vi "Task 9 basic VI.vi"(0 "AE State":T2=enum."Open camera", 1 "error in (no error)":errorcluster) -> (2 "State done?":bool, 3 "Colour output boolean cluster":T1, 4 "error out":errorcluster)   [LabVIEW 2018]
uses:
  Task 9 Sates.ctl
  Modified webcam FGV/Webcam AE.ctl
  <vilib>/userdefined/High Color/IMAQdx.ctl
  I2C Master VI/Arduino_Interfacing.ctl
  I2C Master VI/I2C_MASTER_WRITE_NEW Type Def.ctl
  Elasped Timer/Elapsed timer control.ctl
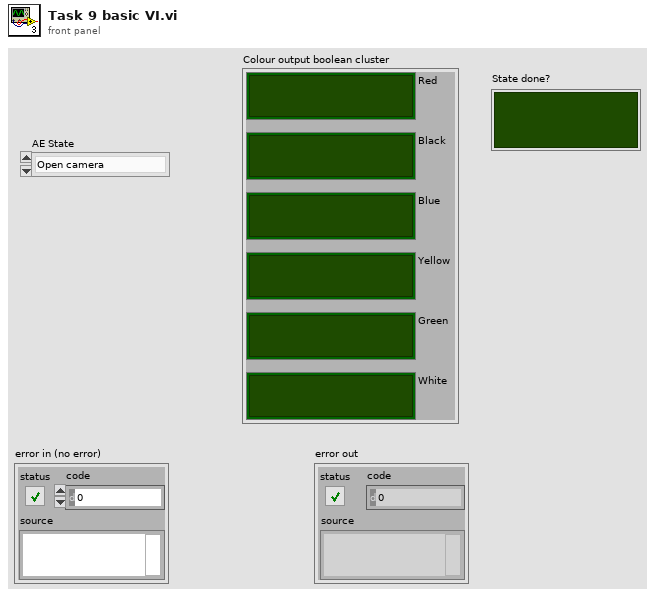
[diagram p1: front panel]
types:
  T1 = cluster{"Red":bool, "Black":bool, "Blue":bool, "Yellow":bool, "Green":bool, "White":bool}
  T2 = typedef "Task 9 Sates.ctl" = enum16{"Initialize", "Open camera", "Move Arm", "Set timer", "Capture images", "Close camera", "Process colour", "Dispose camera buffer"}
  T3 = typedef "Webcam AE.ctl" = enum16{"Initialize Camera", "Open Camera", "Continuous Acquisition", "Close Camera", "Retrieve Image", "Dispose Camera Image Buffer"}
  T4 = typedef "IMAQdx.ctl" = refnum<k21>
  T5 = typedef "I2C_MASTER_WRITE_NEW Type Def.ctl" = enum16{"Ultrasonic sensors", "Stepper origin", "zStepper 13.3k", "zStepper 13k", "zStepper 12k", "zStepper 11k", "zStepper 10k", "zStepper 9k", "zStepper 8k", "zStepper 7k", "zStepper 6k", "zStepper 5k", "zStepper 4k", "zStepper 3k", "zStepper 2k", "zStepper 1k", "zStepper 900", "zStepper 800", "zStepper 700", "zStepper 600", "zStepper 500", "zStepper 400", "zStepper 300", "zStepper 200", "zStepper 100", "zStepper 0", "yStepper control", "Open Claw", "Close Claw", "Soft Reset"}
  T6 = typedef "Arduino_Interfacing.ctl" = enum16{"Initialize", "Write to Arduino", "Read From Arduino"}
  T7 = typedef "Elapsed timer control.ctl" = enum16{"Start", "Pause", "Initialize"}
  T8 = cluster{"Arduino State":u8, "Rotary Switch":u8, "PING A":u8, "PING B":u8, "PING C":u8, "PING D":u8, "y Stepper Position":u8, "z Stepper Position":u8, "Data Out[8]":u8}
  T9 = typedef "IMAQ Image.ctl" = refnum<image>
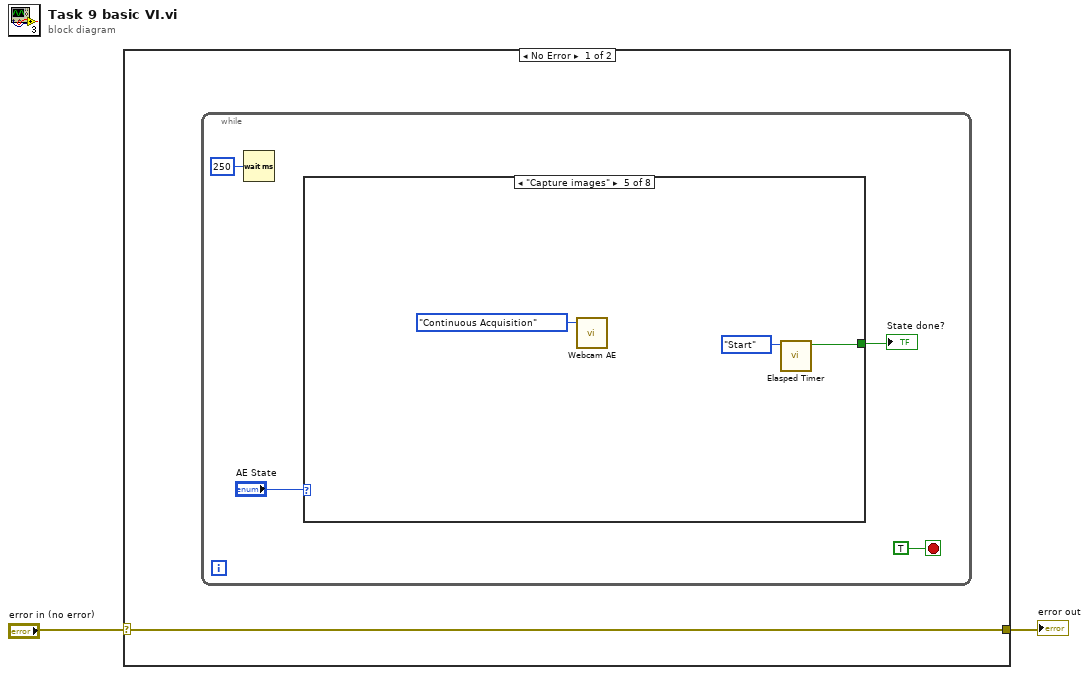
[diagram p0: block diagram]
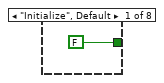
[diagram p2: hidden frame]
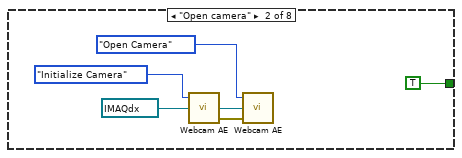
[diagram p3: hidden frame]
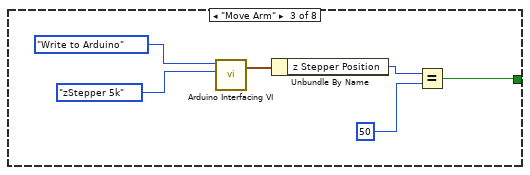
[diagram p4: hidden frame]
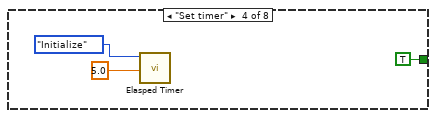
[diagram p5: hidden frame]
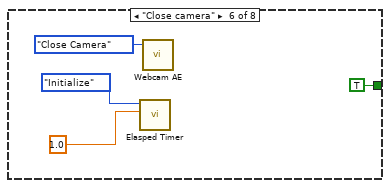
[diagram p6: hidden frame]
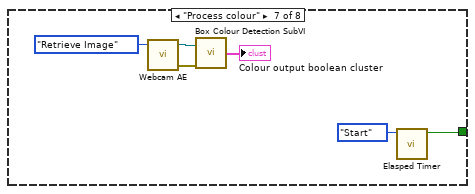
[diagram p7: hidden frame]
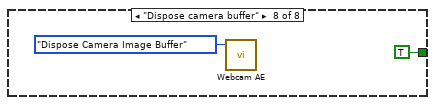
[diagram p8: hidden frame]
diagram:
  n1 = case shown="No Error" "error in (no error)" {
    selector: "error in (no error)" -> [w3 w39]
    tunnel: [w3 w39] -> w1
    frame No Error {
      n2 = while {
        stop <- TRUE stop-if-true
        n3 = Wait (ms)(milliseconds to wait=u32 250) -> ()  [unwired: 1 out]
        n4 = case shown="\"Capture images\"" "AE State" {
          tunnel: [FALSE TRUE w15 TRUE w24 TRUE ("Time Out?!") w31 TRUE ("Time Out?!")] -> w5
          frame "Initialize", Default {
          }
          frame "Open camera" {
            n5 = call "Webcam AE.vi"("Session In"=T4 "cam1", "Camera states"=Webcam_AE."Initialize Camera") -> ("error out"=w14:errorcluster, "Session Out"=w13:T4)  [unwired: 1 in, 1 out]
            n6 = call "Webcam AE.vi"("error in (no error)"=w14, "Session In"=w13, "Camera states"=Webcam_AE."Open Camera") -> ()  [unwired: 3 out]
          }
          frame "Move Arm" {
            n7 = call "Arduino Interfacing VI.vi"("Data to Write"=I2C_MASTER_WRITE_NEW_Type_Def."zStepper 5k", "AE Mode"=Arduino_Interfacing."Write to Arduino") -> ("Arduino Data"=w18:T8)  [unwired: 2 in, 1 out]
            n8 = Unbundle By Name(w18) -> ("z Stepper Position"=w17:u8)
            n9 = Equal?(x=w17, y=u8 50) -> (x = y?=w15:bool)
          }
          frame "Set timer" {
            n10 = call "Elasped Timer.vi"("Time Setting"=5.0, "Action"=Elapsed_timer_control."Initialize") -> ()  [unwired: 6 in, 4 out]
          }
          frame "Capture images" {
            n11 = call "Webcam AE.vi"("Camera states"=Webcam_AE."Continuous Acquisition") -> ()  [unwired: 2 in, 3 out]
            n12 = call "Elasped Timer.vi"("Action"=Elapsed_timer_control."Start") -> ("Time Out?!"=w24:bool)  [unwired: 7 in, 3 out]
          }
          frame "Close camera" {
            n13 = call "Elasped Timer.vi"("Time Setting"=1.0, "Action"=Elapsed_timer_control."Initialize") -> ()  [unwired: 6 in, 4 out]
            n14 = call "Webcam AE.vi"("Camera states"=Webcam_AE."Close Camera") -> ()  [unwired: 2 in, 3 out]
          }
          frame "Process colour" {
            n15 = call "Webcam AE.vi"("Camera states"=Webcam_AE."Retrieve Image") -> ("error out"=w33:errorcluster, "Image Out"=w34:T9)  [unwired: 2 in, 1 out]
            n16 = call "Box Colour Detection SubVI.vi"("Image In"=w34, "Error In"=w33) -> ("Colour output boolean cluster"=→"Colour output boolean cluster":T1)  [unwired: 2 out]
            n17 = call "Elasped Timer.vi"("Action"=Elapsed_timer_control."Start") -> ("Time Out?!"=w31:bool)  [unwired: 7 in, 3 out]
          }
          frame "Dispose camera buffer" {
            n18 = call "Webcam AE.vi"("Camera states"=Webcam_AE."Dispose Camera Image Buffer") -> ()  [unwired: 2 in, 3 out]
          }
        }
        "State done?" <- w5
      }
    }
    frame Error {
    }
  }
  "error out" <- w1
